vi "Pneumatic_Command_Get.vi"   [LabVIEW 2015]
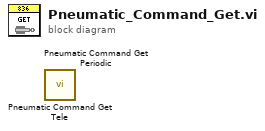
[diagram p0: block diagram]
diagram:
  n1 = call <userlib>:"Pneumatic Command Get Tele.vi"() -> ()  [unwired: 10 in, 2 out]
  n2 = call <userlib>:"Pneumatic Command Get Periodic.vi"() -> ()  [unwired: 10 in, 2 out]
